vi "promedio.vi"() -> ()   [LabVIEW 2021]
panel:
  out "Waveform Chart":dbl(graph)
  out "number (0 to 1)":dbl format="%#_4g"
  in  "stop":bool
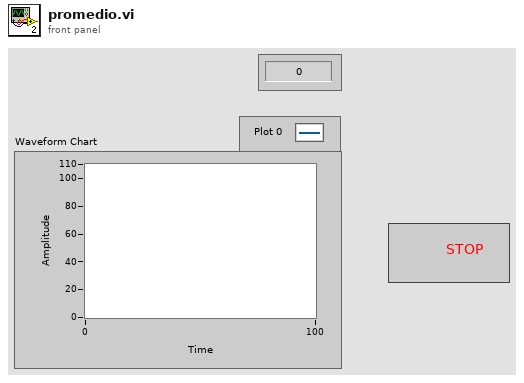
[diagram p1: front panel]
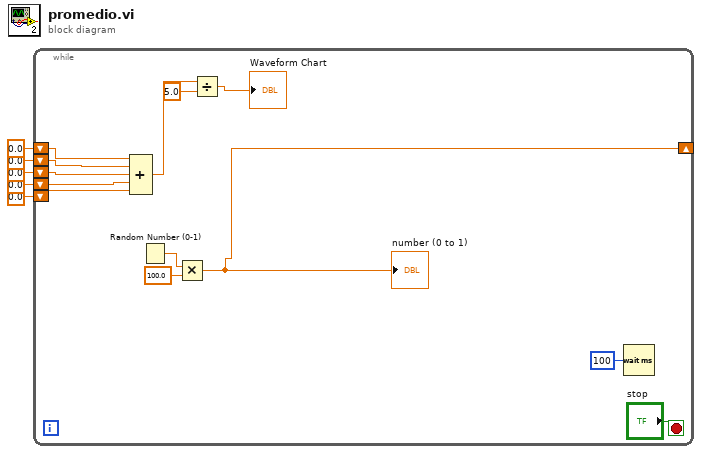
[diagram p0: block diagram]
diagram:
  n1 = while {
    shift-right: [w6] -> _
    shift-left: 0.0 -> [w14]
    shift-left: 0.0 -> [w13]
    shift-left: 0.0 -> [w12]
    shift-left: 0.0 -> [w11]
    shift-left: 0.0 -> [w10]
    stop <- "stop" stop-if-true
    n2 = Compound Arithmetic op=ADD(w14, w13, w12, w11, w10) -> (w9:dbl)
    n3 = Random Number (0-1)() -> (number: 0 to 1=w16:dbl)
    n4 = Multiply(x=w16, y=100.0) -> (x*y=w6:dbl)
    "number (0 to 1)" <- w6
    n5 = Divide(x=w9, y=5.0) -> (x/y=→"Waveform Chart":dbl)
    n6 = Wait (ms)(milliseconds to wait=u32 100) -> ()  [unwired: 1 out]
  }
